vi "beads_DAQ.vi"() -> ()   [LabVIEW 2018]
panel:
  in  "Set Leak":bool
  out "apparent_leak_rate":dbl=4.1159226100440096e-09
  in  "desired_leak_rate (torr*l/s)":dbl format="%.2e"
  out "P_baratron [torr]":dbl=0.00019027336449776468 format="%#_3g"
  out "P_pirani [torr]":dbl=8.903189712596745e-05 format="%#_3g"
  out "P_1Tbaratro [torr]":dbl=0.00035451310561098896 format="%#_3g"
  out "T_elec_rack [C]":dbl
  out "T_opt_table [C]":dbl
  in  "Read pressures?":bool=TRUE
  in  "Read temps?":bool
  in  "img_cluster":cluster{"Take Pic?":bool, "Only Images":bool}
  in  "Picomotor Stepping":T1
  in  "signal type":T2(ring)
  in  "Add small amp?":bool
  in  "Small amp freq (Hz)":dbl=10.0 format="%0.2p"
  in  "Small amp":dbl=1.0 format="%0.2p"
  in  "Flash lamp\n settings:":T3={"Flash lamp?"=FALSE, "Number of cyles\nbetween flashes"=3, "# Pulses"=3, "Stop flashing \nbelow thresh?"=TRUE, "Stop threshold"=15.0, "Pulse voltage?"=FALSE, "Pulse length (ms)"=0.001, "Pulse amp (V)"=0.001}
  in  "Stage settings:":T4={"Set stage?"=FALSE, "start X (um)"=40.0, "stop X (um) "=40.0, "# X Steps"=1, "start Y (um)"=40.0, "stop Y (um) "=40.0, "# Y steps"=1, "start Z (um)"=80.0, "stop Z (um)"=80.0, "# Z steps "=1, "Swp X?"=FALSE, "Amplitude X (um)"=40.0, "Frequency X (Hz)"=10.0, "Amplitude Y (um)"=40.0, "Frequency Y (Hz)"=3.7, "Amplitude Z (um)"=10.0, "Frequency Z (Hz)"=17.0, "Swp Y?"=FALSE, "Swp Z?"=FALSE}
  in  "Electrode settings:":T5={"DC volts (V):\n"=[0.0, 0.0, 0.0, 0.0, 0.0, 0.0, 0.0, 0.0], "Electrode to sweep:"=3, "start volt (V)"=2.0, "stop volt (V) "=2.0, "# V Steps"=1, "start freq (Hz)"=41.0, "stop freq (Hz) "=41.0, "# F steps"=1, "start DC (V)"=0.0, "stop DC (V)"=0.0, "# DC steps "=1, "Digitize electrode\ndrives?"=TRUE, "Sweep electrode?"=TRUE, "Add 0.5*V DC \noffset for amp?"=FALSE, "Use electrode \nconfig file?"=FALSE, "Path"=path "C:/GitHub/opt_lev/labview/DAQ_settings/electrode_sweep.txt", "Use arbitrary\nforce func?"=FALSE, "Voltage vs pos file"=path "C:/GitHub/opt_lev/labview/DAQ_settings/electrode_sweep.txt", "Use Arbitray\nelec drive"=FALSE, "Elec Drive File"=path "C:/GitHub/opt_lev_controls/labview/DAQ_settings/freq_comb_elec3_10V_1-600Hz_nocutsamp.txt", "Filter Elecs?"=FALSE, "Filter Cantilever?"=FALSE, "Control DDS"=TRUE}
  in  "DC supply settings:":T6
  in  "Synth settings:":T7={"start volt (V)"=1.0, "stop volt (V) "=1.0, "# V Steps"=1, "start freq (Hz)"=2000.0, "stop freq (Hz) "=2000.0, "# F steps"=1, "dc offset?"=FALSE, "start DC (V)"=0.5, "stop DC (V)"=0.5, "# DC steps "=1, "Set synth\n(HP33120A)?"=FALSE, "Use arbitrary\nwaveform?"=FALSE, "Arb waveform name:"=""}
  out "Data":dbl[][](graph)
  out "Curr threshold":dbl
  in  "Number of Samples":i32=20000
  in  "Sample Rate [Hz]":dbl=5000.0
  out "Actual Sample \nRate":dbl=5000.0 format="%0.2f"
  in  "Delay between files [s]":dbl=3.0 caption="Delay Time (s)"
  in  "Num files":i32=1000
  in  "File base name":string="turbombar_powfb_xyzcool"
  in  "Directory path":path=path "D:/data/20190626/bead1/spinning/pramp/SF6/rga/discharge_main"
  # "Logging Settings"
  # "Environment"
  # "Picomotor Stepping"
  # "Flash Lamp Settings"
  # "1: -35, 2: -30\n\n1: 32  2: 30"
  # "0"
  # "1"
  # "2"
  # "3"
  # "4"
  # "5"
  # "6"
  # "7"
  # "Acquired Data"
  # "Timing Settings"
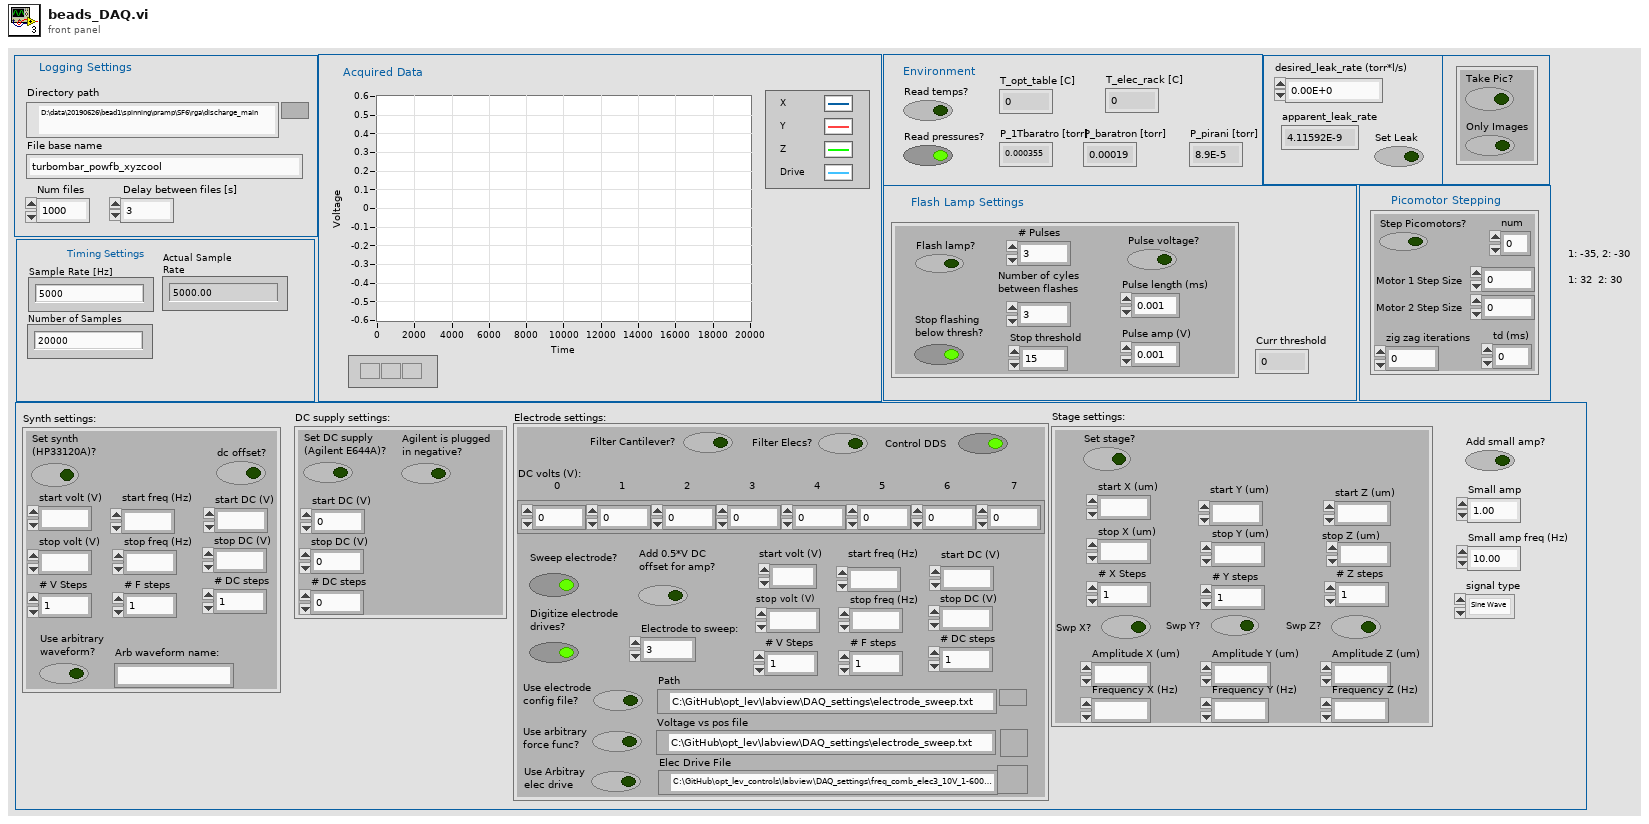
[diagram p1: front panel]
types:
  T1 = cluster{"Motor 1 Step Size":i32, "zig zag iterations":i32, "Motor 2 Step Size":i32, "Step Picomotors?":bool, "td (ms)":dbl, "num":i32}
  T2 = enum16{"Sine Wave", "Triangle Wave", "Square Wave", "Sawtooth Wave"}
  T3 = cluster{"Flash lamp?":bool, "Number of cyles\nbetween flashes":i32, "# Pulses":i32, "Stop flashing \nbelow thresh?":bool, "Stop threshold":dbl, "Pulse voltage?":bool, "Pulse length (ms)":dbl, "Pulse amp (V)":dbl}
  T4 = cluster{"Set stage?":bool, "start X (um)":ext, "stop X (um) ":ext, "# X Steps":i32, "start Y (um)":ext, "stop Y (um) ":ext, "# Y steps":i32, "start Z (um)":ext, "stop Z (um)":ext, "# Z steps ":i32, "Swp X?":bool, "Amplitude X (um)":ext, "Frequency X (Hz)":ext, "Amplitude Y (um)":ext, "Frequency Y (Hz)":ext, "Amplitude Z (um)":ext, "Frequency Z (Hz)":ext, "Swp Y?":bool, "Swp Z?":bool}
  T5 = cluster{"DC volts (V):\n":dbl[], "Electrode to sweep:":i32, "start volt (V)":ext, "stop volt (V) ":ext, "# V Steps":i32, "start freq (Hz)":ext, "stop freq (Hz) ":ext, "# F steps":i32, "start DC (V)":ext, "stop DC (V)":ext, "# DC steps ":i32, "Digitize electrode\ndrives?":bool, "Sweep electrode?":bool, "Add 0.5*V DC \noffset for amp?":bool, "Use electrode \nconfig file?":bool, "Path":path, "Use arbitrary\nforce func?":bool, "Voltage vs pos file":path, "Use Arbitray\nelec drive":bool, "Elec Drive File":path, "Filter Elecs?":bool, "Filter Cantilever?":bool, "Control DDS":bool}
  T6 = cluster{"start DC (V)":ext, "stop DC (V)":ext, "# DC steps ":i32, "Set DC supply\n(Agilent E644A)? ":bool, "Agilent is plugged \nin negative?":bool}
  T7 = cluster{"start volt (V)":ext, "stop volt (V) ":ext, "# V Steps":i32, "start freq (Hz)":ext, "stop freq (Hz) ":ext, "# F steps":i32, "dc offset?":bool, "start DC (V)":ext, "stop DC (V)":ext, "# DC steps ":i32, "Set synth\n(HP33120A)?":bool, "Use arbitrary\nwaveform?":bool, "Arb waveform name:":string}
  T8 = cluster{"Tot Synth Arr":dbl[], "Tot DC Arr":dbl[], "Tot Electrode Arr":dbl[], "Tot Stage Arr":dbl[]}[]
  T9 = cluster{"dup VISA session":refnum<visa-resource-name>, "error out":errorcluster, "task out":refnum<k21>, "error out":errorcluster}
  T10 = cluster{"CmdLib Out":refnum<k24>, "DeviceKey Out":string, "Device Address":i32, "error out":errorcluster}
  T11 = cluster{"Picomotor Instr":cluster{"CmdLib Out":refnum<k24>, "DeviceKey Out":string, "Device Address":i32, "error out":errorcluster}, "Picomotor Stepping":cluster{"Motor 1 Step Size":i32, "zig zag iterations":i32, "Motor 2 Step Size":i32, "Step Picomotors?":bool, "td (ms)":dbl, "num":i32}}
  T12 = cluster{"Number of Samples":i32, "Sample Rate [Hz]":dbl, "Physical Channels (Position signals)":tag, "Physical Channel (drive signals)":tag, "Sample Clock Source":tag, "Physical Channel (drive signals)":tag}
  T13 = enum16{"open", "replace", "create", "open or create", "replace or create", "replace or create with confirmation"}
  T14 = cluster{"CmdLib Out":refnum<k24>, "DeviceKey Out":string, "Device Address Out":i32, "error out":errorcluster, "Step Picomotors?":bool}
  T15 = cluster{"appended path":path, "base_path":path, "filename":string}
  T16 = cluster{"Output channel (for flashing)":tag, i32, "path out":path, "Flash lamp\n settings:":cluster{"Flash lamp?":bool, "Number of cyles\nbetween flashes":i32, "# Pulses":i32, "Stop flashing \nbelow thresh?":bool, "Stop threshold":dbl, "Pulse voltage?":bool, "Pulse length (ms)":dbl, "Pulse amp (V)":dbl}}
  T17 = cluster{"dup VISA session":refnum<visa-resource-name>, "error out":errorcluster, "Agilent is \nplugged in \nnegative?":bool, "electrodes task":refnum<k21>, "electrodes task error":errorcluster, "Set synth":bool, "Set DC":bool}
  T18 = cluster{"task out":refnum<k21>, "error out":errorcluster, "task out":refnum<k21>, "error out":errorcluster, "task out":refnum<k21>, "error out":errorcluster, "SampClk.Rate":dbl}
  T19 = cluster{"task out":refnum<k21>, "error out":errorcluster, "task out":refnum<k21>, "error out":errorcluster, "trigger task":refnum<k21>, "trigger task error":errorcluster}
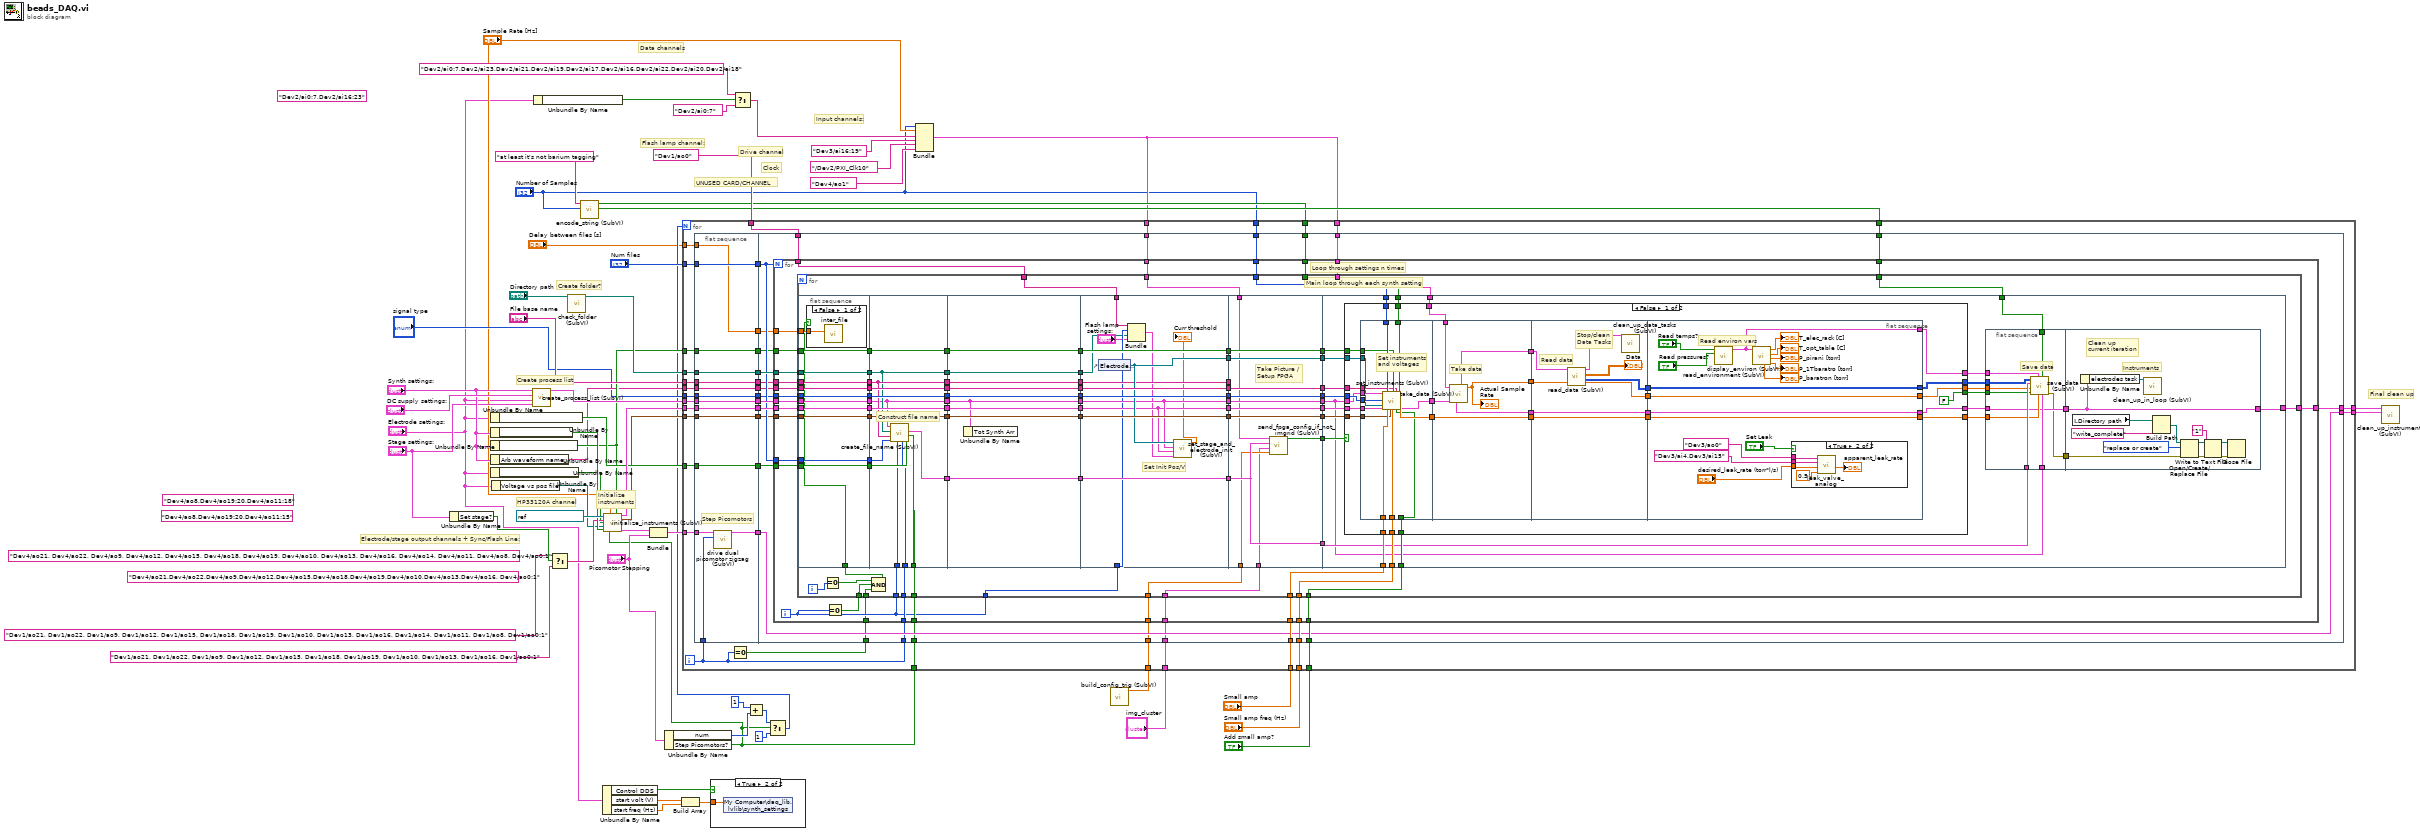
[diagram p0: block diagram]
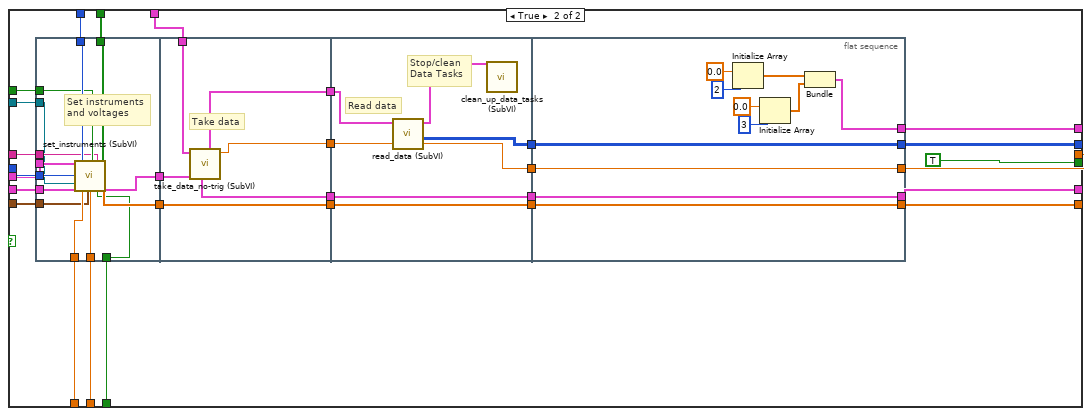
[diagram p5: hidden frame]
diagram:
  (unwired) tag "Dev4/ao21, Dev4/ao22, Dev4/ao9, Dev4/ao12, Dev4/ao15, Dev4/ao18, Dev4/ao19, Dev4/ao10, Dev4/ao13, Dev4/ao16, Dev4/ao14, Dev4/ao11, Dev4/ao8, Dev4/ao0:1" ("Output channel (for flashing)")
  (unwired) tag "Dev4/ao21,Dev4/ao22,Dev4/ao9,Dev4/ao12,Dev4/ao15,Dev4/ao18,Dev4/ao19,Dev4/ao10,Dev4/ao13,Dev4/ao16, Dev4/ao0:1" ("Output channel (for flashing)")
  (unwired) tag "Dev4/ao8,Dev4/ao19:20,Dev4/ao11:18" ("Output channel (for flashing)")
  (unwired) tag "Dev2/ai0:7,Dev2/ai16:23" ("Physical Channels (Position signals)")
  (unwired) tag "Dev4/ao8,Dev4/ao19:20,Dev4/ao11:15" ("Output channel (for flashing)")
  # "Final clean up"
  # "Clock"
  # "Drive channel"
  # "UNUSED CARD/CHANNEL"
  # "Data channels"
  # "Initialize\ninstruments"
  # "Electrode/stage output channels + Sync/Flash Line:"
  # "HP33120A channel"
  # "Flash lamp channel:"
  # "Create process list"
  # "Input channels:"
  # "Create folder?"
  n1 = Unbundle By Name("Stage settings:") -> ("Set stage?"=w42:bool)
  n2 = Unbundle By Name("Synth settings:") -> ("Use arbitrary\nwaveform?"=w36:bool)
  n3 = Unbundle By Name("Electrode settings:") -> ("Use electrode \nconfig file?"=w40:bool)
  n4 = Unbundle By Name("Synth settings:") -> ("Set synth\n(HP33120A)?"=w54:bool)
  n5 = Unbundle By Name("Synth settings:") -> ("Arb waveform name:"=w35:string)
  n6 = Unbundle By Name("Electrode settings:") -> ("Use arbitrary\nforce func?"=w33:bool)
  n7 = Unbundle By Name("Electrode settings:") -> ("Voltage vs pos file"=w32:path)
  n8 = call "create_process_list (SubVI).vi"("Synth settings:"="Synth settings:", "DC supply settings:"="DC supply settings:", "Electrode settings:"="Electrode settings:", "Stage settings:"="Stage settings:") -> ("Process list"=w57:T8)  [unwired: 5 in]
  n9 = Unbundle By Name("Electrode settings:") -> ("Digitize electrode\ndrives?"=w45:bool)
  n10 = Select(t=tag "Dev1/ao21, Dev1/ao22, Dev1/ao9, Dev1/ao12, Dev1/ao15, Dev1/ao18, Dev1/ao19, Dev1/ao10, Dev1/ao13, Dev1/ao16, Dev1/ao14, Dev1/ao11, Dev1/ao8, Dev1/ao0:1" ("Output channel (for flashing)"), s=w42, f=tag "Dev1/ao21, Dev1/ao22, Dev1/ao9, Dev1/ao12, Dev1/ao15, Dev1/ao18, Dev1/ao19, Dev1/ao10, Dev1/ao13, Dev1/ao16, Dev1/ao0:1" ("Output channel (for flashing)")) -> (s? t:f=w41:tag)
  n11 = call "check_folder (SubVI).vi"("path in"="Directory path") -> ("path out"=w56:path)  [unwired: 10 in]
  n12 = call "encode_string (SubVI).vi"("nsamp"="Number of Samples", "encode_string"="at least it's not barium tagging") -> ("encoded_cropped"=w14:bool[], "encoded_out"=w12:bool[])  [unwired: 8 in]
  n13 = Unbundle By Name("Electrode settings:") -> ("Control DDS"=w4:bool, "start volt (V)"=w3:ext, "start freq (Hz)"=w2:ext)
  n14 = Unbundle By Name("Picomotor Stepping") -> ("num"=w20:i32, "Step Picomotors?"=w18:bool)
  n15 = call "initialize_instruments (SubVI).vi"("VISA Refnum in"=refnum<visa-resource-name> "GPIB0::11::INSTR" ("VISA session"), "Sample rate"="Sample Rate [Hz]", "trig_wfm"=w36, "Electrode outupt channels"=w41, "make volt file"=w33, "volt file path"=w32, "Use synth?"=w54, "Step Picomotors?"=w18) -> ("instrument config"=w53:T9, "Volt vs pos array"=w31:cluster{dbl, dbl}[], "Picomotor Instr"=w25:T10)  [unwired: 5 in]
  n16 = Bundle("Picomotor Instr"=w25, "Picomotor Stepping"="Picomotor Stepping") -> (w24:T11)  [unwired: 1 in]
  n17 = Build Array(w3, w2) -> (w1:ext[])
  n18 = case shown="True" w4 {
    tunnel: w1 -> [_ w59]
    frame False {
    }
    frame True {
      n19 = shared-variable "My Computer\\daq_lib.lvlib\\synth_settings"(w59) -> ()  [unwired: 1 in, 1 out]
    }
  }
  n20 = Select(t=tag "Dev2/ai0:7,Dev2/ai23,Dev2/ai21,Dev2/ai19,Dev2/ai17,Dev2/ai16,Dev2/ai22,Dev2/ai20,Dev2/ai18" ("Physical Channels (Position signals)"), s=w45, f=tag "Dev2/ai0:7" ("Physical Channels (Position signals)")) -> (s? t:f=w43:tag)
  n21 = Add(x=1, y=w20) -> (x+y=w19:i32)
  n22 = Select(t=w19, s=w18, f=1) -> (s? t:f=w23:i32)
  n23 = Bundle("Number of Samples"="Number of Samples", "Sample Rate [Hz]"="Sample Rate [Hz]", "Physical Channels (Position signals)"=w43, "Physical Channel (drive signals)"=tag "Dev3/ai16:19", "Sample Clock Source"=tag "/Dev2/PXI_Clk10", "Physical Channel (drive signals)"=tag "Dev4/ao1") -> (w11:T12)  [unwired: 1 in]
  n24 = call "build_config_trig (SubVI).vi"() -> ("config_trig"=w10:dbl[])  [unwired: 11 in]
  n25 = for {
    N: w23 -> [_]
    tunnel: w57 -> [w99]
    tunnel: w56 -> [w98]
    tunnel: w53 -> [w97]
    tunnel: "Num files" -> [w96]
    tunnel: "File base name" -> [w95]
    tunnel: w11 -> [w94]
    tunnel: [w93] -> w47
    tunnel: "Number of Samples" -> [w92]
    tunnel: w40 -> [w91]
    tunnel: "Small amp" -> [w90]
    tunnel: "Small amp freq (Hz)" -> [w89]
    tunnel: "Add small amp?" -> [w88]
    tunnel: w36 -> [w87]
    tunnel: w35 -> [w86]
    tunnel: w31 -> [w85]
    tunnel: tag "Dev1/ao0" ("Output channel (for flashing)") -> [w84]
    tunnel: "signal type" -> [w83]
    tunnel: [w81] -> w27
    tunnel: w24 -> [w82]
    tunnel: w18 -> [w69]
    tunnel: "img_cluster" -> [w68]
    tunnel: w14 -> [w67]
    tunnel: "Delay between files [s]" -> [w65]
    tunnel: w12 -> [w64]
    tunnel: w11 -> [w63]
    tunnel: w10 -> [w62]
    i -> [w61]
    n26 = flat-sequence {
      tunnel: w82 -> [w103]
      tunnel: w83 -> [w104]
      tunnel: w85 -> [w105]
      tunnel: w86 -> [w106]
      tunnel: w87 -> [w107]
      tunnel: w91 -> [w108]
      tunnel: w95 -> [w109]
      tunnel: w96 -> [w110]
      tunnel: w97 -> [w111]
      tunnel: w98 -> [w112]
      tunnel: w99 -> [w113]
      tunnel: [w113] -> w80
      tunnel: [w112] -> w79
      tunnel: [w111] -> w78
      tunnel: [w110] -> w77
      tunnel: [w109] -> w76
      tunnel: [w108] -> w75
      tunnel: [w107] -> w74
      tunnel: [w106] -> w73
      tunnel: [w105] -> w72
      tunnel: [w104] -> w71
      tunnel: [w102] -> w70
      tunnel: w61 -> [w101]
      tunnel: [w100] -> w66
      tunnel: w65 -> [w100]
      tunnel: w94 -> [w135]
      tunnel: [w134] -> w93
      tunnel: w92 -> [w133]
      tunnel: w90 -> [w131]
      tunnel: w89 -> [w130]
      tunnel: w88 -> [w129]
      tunnel: w84 -> [w125]
      tunnel: [w123] -> w81
      tunnel: w80 -> [w140]
      tunnel: w79 -> [w139]
      tunnel: w78 -> [w138]
      tunnel: w77 -> [w137]
      tunnel: w76 -> [w136]
      tunnel: w75 -> [w132]
      tunnel: w74 -> [w128]
      tunnel: w73 -> [w127]
      tunnel: w72 -> [w126]
      tunnel: w71 -> [w124]
      tunnel: w70 -> [w123]
      tunnel: w61 -> [w122]
      tunnel: w69 -> [w121]
      tunnel: w68 -> [w120]
      tunnel: w67 -> [w119]
      tunnel: w66 -> [w118]
      tunnel: w64 -> [w117]
      tunnel: w63 -> [w116]
      tunnel: w62 -> [w115]
      tunnel: w60 -> [w114]
      frame #0 {
        # "Step Picomotors"
        n27 = call "drive dual picomotor zigzag (SubVI).vi"("Picomotor Index"=w101, "Picomotor Cluster"=w103) -> ("Picomotor Instr Out"=w102:T14)  [unwired: 9 in]
      }
      frame #1 {
        n28 = for {
          N: w137 -> [_]
          tunnel: w140 -> [w168]
          tunnel: w125 -> [w146]
          tunnel: w139 -> [w167]
          tunnel: w138 -> [w166]
          tunnel: w137 -> [w165]
          tunnel: w136 -> [w164]
          tunnel: w135 -> [w163]
          tunnel: [w162] -> w134
          tunnel: w133 -> [w161]
          tunnel: w132 -> [w160]
          tunnel: w131 -> [w159]
          tunnel: w130 -> [w158]
          tunnel: w129 -> [w157]
          tunnel: w128 -> [w156]
          tunnel: w127 -> [w155]
          tunnel: w126 -> [w154]
          tunnel: w124 -> [w153]
          tunnel: w122 -> [w152]
          tunnel: w121 -> [w151]
          tunnel: w120 -> [w150]
          tunnel: w119 -> [w149]
          tunnel: w118 -> [w148]
          tunnel: w117 -> [w147]
          tunnel: w116 -> [w145]
          tunnel: w115 -> [w144]
          tunnel: w114 -> [w141]
          i -> [w143]
          # "Loop through settings n times"
          n29 = Equal To 0?(x=w143) -> (x = 0?=w142:bool)
          n30 = for {
            tunnel: w168 -> [w231] mode=indexing
            tunnel: w167 -> [w246]
            tunnel: w166 -> [w245]
            tunnel: w165 -> [w244]
            tunnel: w164 -> [w243]
            tunnel: w163 -> [w242]
            tunnel: [w241] -> w162
            tunnel: w161 -> [w240]
            tunnel: w160 -> [w239]
            tunnel: w159 -> [w238]
            tunnel: w158 -> [w237]
            tunnel: w157 -> [w236]
            tunnel: w156 -> [w235]
            tunnel: w155 -> [w234]
            tunnel: w154 -> [w233]
            tunnel: w153 -> [w232]
            tunnel: w152 -> [w211]
            tunnel: w151 -> [w210]
            tunnel: w143 -> [w212]
            tunnel: w150 -> [w188]
            tunnel: w149 -> [w213]
            tunnel: w148 -> [w199]
            tunnel: w147 -> [w198]
            tunnel: w146 -> [w197]
            tunnel: w143 -> [w196]
            tunnel: w145 -> [w195]
            tunnel: w144 -> [w169]
            tunnel: w142 -> [w192]
            tunnel: w141 -> [w191]
            i -> [w194]
            # "Main loop through each synth setting"
            n31 = flat-sequence {
              tunnel: w232 -> [w249]
              tunnel: w233 -> [w250]
              tunnel: w234 -> [w251]
              tunnel: w235 -> [w252]
              tunnel: w239 -> [w253]
              tunnel: w243 -> [w254]
              tunnel: w244 -> [w255]
              tunnel: w245 -> [w256]
              tunnel: w246 -> [w257]
              tunnel: w231 -> [w258]
              tunnel: [w258] -> w209
              tunnel: [w257] -> w208
              tunnel: [w256] -> w207
              tunnel: [w255] -> w206
              tunnel: [w254] -> w205
              tunnel: [w253] -> w204
              tunnel: [w252] -> w203
              tunnel: [w251] -> w202
              tunnel: [w250] -> w201
              tunnel: [w249] -> w200
              tunnel: w199 -> [w248]
              tunnel: w190 -> [w247]
              tunnel: [w266] -> w187
              tunnel: [w267] -> w185
              tunnel: [w273] -> w183
              tunnel: [w268] -> w181
              tunnel: [w272] -> w179
              tunnel: [w271] -> w177
              tunnel: [w270] -> w175
              tunnel: [w269] -> w173
              tunnel: [w260] -> w171
              tunnel: w212 -> [w263]
              tunnel: w211 -> [w262]
              tunnel: w210 -> [w261]
              tunnel: w209 -> [w266]
              tunnel: w208 -> [w267]
              tunnel: w207 -> [w273]
              tunnel: w206 -> [w265]
              tunnel: w205 -> [w268]
              tunnel: w204 -> [w264]
              tunnel: w203 -> [w272]
              tunnel: w202 -> [w271]
              tunnel: w201 -> [w270]
              tunnel: w200 -> [w269]
              tunnel: w187 -> [w274]
              tunnel: [w274] -> w186
              tunnel: w185 -> [w282]
              tunnel: [w282] -> w184
              tunnel: w183 -> [w281]
              tunnel: [w281] -> w182
              tunnel: w181 -> [w280]
              tunnel: [w280] -> w180
              tunnel: w179 -> [w279]
              tunnel: [w279] -> w178
              tunnel: w177 -> [w278]
              tunnel: [w278] -> w176
              tunnel: w175 -> [w277]
              tunnel: [w277] -> w174
              tunnel: w173 -> [w276]
              tunnel: [w276] -> w172
              tunnel: w171 -> [w275]
              tunnel: [w275] -> w170
              tunnel: [w292] -> w230
              tunnel: [w291] -> w228
              tunnel: [w297] -> w226
              tunnel: [w296] -> w224
              tunnel: [w295] -> w222
              tunnel: [w294] -> w220
              tunnel: [w293] -> w218
              tunnel: [w290] -> w216
              tunnel: [w289] -> w214
              tunnel: w186 -> [w292]
              tunnel: w184 -> [w286]
              tunnel: w182 -> [w291]
              tunnel: w180 -> [w290]
              tunnel: w178 -> [w297]
              tunnel: w176 -> [w296]
              tunnel: w174 -> [w295]
              tunnel: w172 -> [w294]
              tunnel: w170 -> [w289]
              tunnel: w197 -> [w288]
              tunnel: w196 -> [w287]
              tunnel: w230 -> [w309]
              tunnel: [w309] -> w229
              tunnel: w228 -> [w308]
              tunnel: [w308] -> w227
              tunnel: w226 -> [w307]
              tunnel: [w307] -> w225
              tunnel: w224 -> [w306]
              tunnel: [w306] -> w223
              tunnel: w222 -> [w305]
              tunnel: [w305] -> w221
              tunnel: w220 -> [w304]
              tunnel: [w304] -> w219
              tunnel: w218 -> [w303]
              tunnel: [w303] -> w217
              tunnel: w216 -> [_]
              tunnel: [w301] -> w215
              tunnel: w214 -> [w301]
              tunnel: w195 -> [w302]
              tunnel: w169 -> [w300]
              tunnel: [w298] -> w189
              tunnel: w188 -> [w299]
              tunnel: [w313] -> w241
              tunnel: w242 -> [w334]
              tunnel: w198 -> [w323]
              tunnel: w215 -> [w321]
              tunnel: w217 -> [w324]
              tunnel: w219 -> [w325]
              tunnel: w221 -> [w326]
              tunnel: w223 -> [w327]
              tunnel: w225 -> [w328]
              tunnel: w227 -> [w333]
              tunnel: w229 -> [w320]
              tunnel: w236 -> [w329]
              tunnel: w237 -> [w330]
              tunnel: w238 -> [w331]
              tunnel: w240 -> [w332]
              tunnel: w213 -> [w315]
              tunnel: w189 -> [w322]
              frame #0 {
                n32 = case shown="False" w247 {
                  tunnel: w248 -> [w259 _]
                  frame False {
                    n33 = call "inter_file"("Delay Time (s)"=w259) -> ()  [unwired: 10 in, 1 out]
                  }
                  frame True {
                  }
                }
              }
              frame #1 {
                # "Construct file name"
                n34 = call "create_file_name (SubVI).vi"("Use electrode config?"=w264, "Step Picomotors?"=w261, "picomotor index"=w262, "file_idx"=w263, "num files"=w265, "base name"=w268, "Path"=w267, "Cluster"=w266) -> ("output cluster"=w260:T15)  [unwired: 3 in]
              }
              frame #2 {
                n35 = Unbundle By Name(w274) -> ()  [unwired: 1 out]
              }
              frame #3 {
                # "Set Init Pos/V"
                n36 = control-ref of="Electrode settings:"() -> (w293:refnum<vi>)
                n37 = Bundle("Output channel (for flashing)"=w288, w287, "path out"=w286, "Flash lamp\n settings:"="Flash lamp\n settings:") -> (w284:T16)  [unwired: 1 in]
                n38 = call "set_stage_and_electrode_init (SubVI).vi"("Flash lamp settings:"=w284, "instrument config"=w291, "Process list"=w292, "Cluster in"=w293) -> ("Curr threshold"=→"Curr threshold":dbl)  [unwired: 7 in]
              }
              frame #4 {
                # "Take Picture / \nSetup FPGA"
                n39 = call "send_fpga_config_if_not_imgrid (SubVI).vi"("config_trig"=w300, "img_cluster"=w299, "file_path_cluster"=w301, "channel settings"=w302) -> ("Only Images"=w298:bool)  [unwired: 7 in]
              }
              frame #5 {
                n40 = case shown="False" w322 {
                  tunnel: [w362 w439] -> w314
                  tunnel: w320 -> [w363 w440]
                  tunnel: w334 -> [w372 w449]
                  tunnel: w333 -> [w385 w462]
                  tunnel: w332 -> [w384 w461]
                  tunnel: w331 -> [w383 w460]
                  tunnel: w330 -> [w382 w459]
                  tunnel: w329 -> [w381 w458]
                  tunnel: w328 -> [w380 w457]
                  tunnel: w327 -> [w379 w456]
                  tunnel: w326 -> [w378 w455]
                  tunnel: w325 -> [w377 w454]
                  tunnel: w324 -> [w376 w453]
                  tunnel: w323 -> [w375 w452]
                  tunnel: [w361 w438] -> w319
                  tunnel: [w360 w434] -> w318
                  tunnel: [w359 w437] -> w317
                  tunnel: [w358 w436] -> w316
                  tunnel: [FALSE TRUE] -> w311
                  frame False {
                    n41 = flat-sequence {
                      tunnel: w363 -> [w399]
                      tunnel: w385 -> [w396]
                      tunnel: w384 -> [w395]
                      tunnel: w383 -> [w394]
                      tunnel: w382 -> [w393]
                      tunnel: w381 -> [w392]
                      tunnel: w380 -> [w391]
                      tunnel: w379 -> [w390]
                      tunnel: w378 -> [w389]
                      tunnel: w377 -> [w388]
                      tunnel: w376 -> [w387]
                      tunnel: w375 -> [w386]
                      tunnel: [w398] -> w374
                      tunnel: [w397] -> w373
                      tunnel: w374 -> [w405]
                      tunnel: w373 -> [w403]
                      tunnel: w372 -> [w402]
                      tunnel: [w405] -> w371
                      tunnel: [w404] -> w370
                      tunnel: [w401] -> w369
                      tunnel: [w400] -> w368
                      tunnel: w371 -> [w412]
                      tunnel: w370 -> [w408]
                      tunnel: w369 -> [w411]
                      tunnel: w368 -> [w410]
                      tunnel: [w412] -> w367
                      tunnel: [w411] -> w366
                      tunnel: [w410] -> w365
                      tunnel: [w406] -> w364
                      tunnel: w367 -> [w428]
                      tunnel: w366 -> [w427]
                      tunnel: w365 -> [w426]
                      tunnel: w364 -> [w425]
                      tunnel: [w428] -> w361
                      tunnel: [w427] -> w362
                      tunnel: [w426] -> w358
                      tunnel: [w425] -> w359
                      tunnel: [w417] -> w360
                      frame #0 {
                        # "Set instruments\nand voltages"
                        n42 = call "set_instruments (SubVI).vi"("Process list"=w399, "signal type"=w388, "electrodes reference"=w387, "instrument config"=w396, "Num samples"=w395, "small amp"=w394, "Volt vs pos array"=w389, "wfm?"=w391, "small amp freq"=w393, "User Def. Wfm Name"=w390, "Add small amp?"=w392, "encode_bits"=w386) -> ("DC volts arr"=w398:dbl[], "instrum out"=w397:T17)  [unwired: 6 in]
                      }
                      frame #1 {
                        # "Take data"
                        n43 = call "take_data (SubVI).vi"("instrum in"=w403, "channel settings"=w402) -> ("Actual Sample Rate"=w400:dbl, "data_cluster"=w404:T18, "instrum out"=w401:T17)  [unwired: 7 in]
                        "Actual Sample \nRate" <- w400
                      }
                      frame #2 {
                        # "Read data"
                        # "Stop/clean \nData Tasks"
                        n44 = call "read_data (SubVI).vi"("data tasks"=w408) -> ("Rescaled data"=w406:i16[][], "Output data"=→"Data":dbl[][], "output data tasks"=w407:T19)  [unwired: 7 in, 1 out]
                        n45 = call "clean_up_data_tasks (SubVI).vi"("data tasks"=w407) -> ()  [unwired: 11 in]
                      }
                      frame #3 {
                        # "Read environ vars"
                        n46 = call "read_environment (SubVI).vi"("Read pressures?"="Read pressures?", "Read temps?"="Read temps?") -> ("environ cluster"=w417:cluster{dbl[], dbl[]})  [unwired: 9 in]
                        n47 = call "display_environ (SubVI).vi"("environ cluster"=w417) -> ("P_pirani"=→"P_1Tbaratro [torr]":dbl, "P_cc"=→"P_pirani [torr]":dbl, "T_opt_table"=→"T_opt_table [C]":dbl, "T_elec_rack"=→"T_elec_rack [C]":dbl, "P_baratron"=→"P_baratron [torr]":dbl)  [unwired: 6 in]
                        n48 = case shown="True" "Set Leak" {
                          tunnel: "desired_leak_rate (torr*l/s)" -> [_ w433]
                          tunnel: tag "Dev3/ao0" ("leak_control_channel") -> [_ w432]
                          tunnel: tag "Dev3/ai4,Dev3/ai15" ("valve_pos_channel") -> [_ w431]
                          frame False {
                          }
                          frame True {
                            n49 = call "leak_valve_analog.vi"("read/write delay"=0.5, "desired_leak_rate (torr*l/s)"=w433, "valve_pos_channel"=w431, "leak_control_channel"=w432) -> ("apparent_leak_rate"=→"apparent_leak_rate":dbl)  [unwired: 4 in, 2 out]
                          }
                        }
                      }
                    }
                  }
                  frame True {
                    n50 = flat-sequence {
                      tunnel: w440 -> [w476]
                      tunnel: w462 -> [w473]
                      tunnel: w461 -> [w472]
                      tunnel: w460 -> [w471]
                      tunnel: w459 -> [w470]
                      tunnel: w458 -> [w469]
                      tunnel: w457 -> [w468]
                      tunnel: w456 -> [w467]
                      tunnel: w455 -> [w466]
                      tunnel: w454 -> [w465]
                      tunnel: w453 -> [w464]
                      tunnel: w452 -> [w463]
                      tunnel: [w475] -> w451
                      tunnel: [w474] -> w450
                      tunnel: w451 -> [w482]
                      tunnel: w450 -> [w480]
                      tunnel: w449 -> [w479]
                      tunnel: [w482] -> w448
                      tunnel: [w481] -> w447
                      tunnel: [w478] -> w446
                      tunnel: [w477] -> w445
                      tunnel: w448 -> [w488]
                      tunnel: w447 -> [w485]
                      tunnel: w446 -> [w487]
                      tunnel: w445 -> [w486]
                      tunnel: [w488] -> w444
                      tunnel: [w487] -> w443
                      tunnel: [w486] -> w442
                      tunnel: [w483] -> w441
                      tunnel: w444 -> [w499]
                      tunnel: w443 -> [w498]
                      tunnel: w442 -> [w497]
                      tunnel: w441 -> [w496]
                      tunnel: [w499] -> w438
                      tunnel: [w498] -> w439
                      tunnel: [w497] -> w436
                      tunnel: [w496] -> w437
                      tunnel: [w491] -> w434
                      frame #0 {
                        # "Set instruments\nand voltages"
                        n51 = call "set_instruments (SubVI).vi"("Process list"=w476, "signal type"=w465, "electrodes reference"=w464, "instrument config"=w473, "Num samples"=w472, "small amp"=w471, "Volt vs pos array"=w466, "wfm?"=w468, "small amp freq"=w470, "User Def. Wfm Name"=w467, "Add small amp?"=w469, "encode_bits"=w463) -> ("DC volts arr"=w475:dbl[], "instrum out"=w474:T17)  [unwired: 6 in]
                      }
                      frame #1 {
                        # "Take data"
                        n52 = call "take_data_no-trig (SubVI).vi"("instrum in"=w480, "channel settings"=w479) -> ("Actual Sample Rate"=w477:dbl, "data_cluster"=w481:T18, "instrum out"=w478:T17)  [unwired: 7 in]
                      }
                      frame #2 {
                        # "Read data"
                        # "Stop/clean \nData Tasks"
                        n53 = call "read_data (SubVI).vi"("data tasks"=w485) -> ("Rescaled data"=w483:i16[][], "output data tasks"=w484:T19)  [unwired: 7 in, 2 out]
                        n54 = call "clean_up_data_tasks (SubVI).vi"("data tasks"=w484) -> ()  [unwired: 11 in]
                      }
                      frame #3 {
                        n55 = Initialize Array(0.0 ("element"), 2 ("dimension size")) -> (w490:dbl[])
                        n56 = Initialize Array(0.0 ("element"), 3 ("dimension size")) -> (w489:dbl[])
                        n57 = Bundle(w490, w489) -> (w491:cluster{dbl[], dbl[]})  [unwired: 1 in]
                      }
                    }
                  }
                }
                n58 = flat-sequence {
                  tunnel: w321 -> [w344]
                  tunnel: w320 -> [w343]
                  tunnel: w319 -> [w342]
                  tunnel: w318 -> [w341]
                  tunnel: w317 -> [w340]
                  tunnel: w316 -> [w339]
                  tunnel: w315 -> [w338]
                  tunnel: w314 -> [w337]
                  tunnel: [w337] -> w312
                  tunnel: w311 -> [w336]
                  tunnel: [w335] -> w310
                  tunnel: [w355] -> w313
                  tunnel: w312 -> [w355]
                  tunnel: w310 -> [w354]
                  frame #0 {
                    # "Save data"
                    n59 = call "save_data (SubVI).vi"("Process list"=w343, "encoded_bits"=w338, "DC volts arr"=w342, "environ cluster"=w341, "imgrid"=w336, "Fsamp"=w339, "file_path_cluster"=w344, "data"=w340) -> ("error out"=w335:errorcluster)  [unwired: 3 in]
                  }
                  frame #1 {
                    # "Clean up\ncurrent iteration"
                    # "Instruments"
                    n60 = local read "Directory path"() -> (w353:path)
                    n61 = Unbundle By Name(w355) -> ("electrodes task"=w356:refnum<k21>)
                    n62 = call "clean_up_in_loop (SubVI).vi"("Refnum in"=w356) -> ()  [unwired: 10 in, 1 out]
                    n63 = Build Path(base path=w353, name or relative path="write_complete") -> (appended path=w351:path)
                    n64 = Open/Create/Replace File(file path (use dialog)=w351, error in=w354, operation (0:open)=T13."replace or create") -> (refnum out=w349:refnum<file>, error out=w350:errorcluster)  [unwired: 3 in, 1 out]
                    n65 = Write to Text File(file (use dialog)=w349, text="1", error in=w350) -> (refnum out=w345:refnum<file>, error out=w346:errorcluster)  [unwired: 1 in, 1 out]
                    n66 = Close File(refnum=w345, error in=w346) -> ()  [unwired: 2 out]
                  }
                }
              }
            }
            n67 = Equal To 0?(x=w194) -> (x = 0?=w193:bool)
            n68 = Compound Arithmetic op=AND(w193, w192, w191) -> (w190:bool)
          }
        }
      }
    }
    n69 = Equal To 0?(x=w61) -> (x = 0?=w60:bool)
  }
  n70 = call "clean_up_instruments (SubVI).vi"("Picomotor Instr Out"=w27, "instrum out"=w47) -> ()  [unwired: 10 in]
